vi "Create.vi"(7 "mode settings":variant, 8 "error in":errorcluster, 9 "number of channels":i32, 10 "channel settings":variant, 11 "digital output mode in":refnum<class "Digital Output Mode.lvclass">) -> (0 "error out":errorcluster, 1 "channels":refnum<class "Channel.lvclass">[](array[class]), 3 "digital output mode out":refnum<class "Digital Output Mode.lvclass">)   [LabVIEW 2017, in "Scan Engine Scripting.lvlib" / "Digital Output Mode.lvclass"]
uses:
  Digital Output Mode.lvclass
  Channel Classes/Channel/Channel.lvclass
  Controls/digital channel settings.ctl
  Channel Classes/DO Channel/DO Channel.lvclass
  C:/dev/github.com/debryant/niveristand-scan-engine-ethercat-custom-device/Custom Device Source/Scripting/Modules/Channel Classes/Channel/Channel.lvclass
  Scan Engine Scripting.lvlib
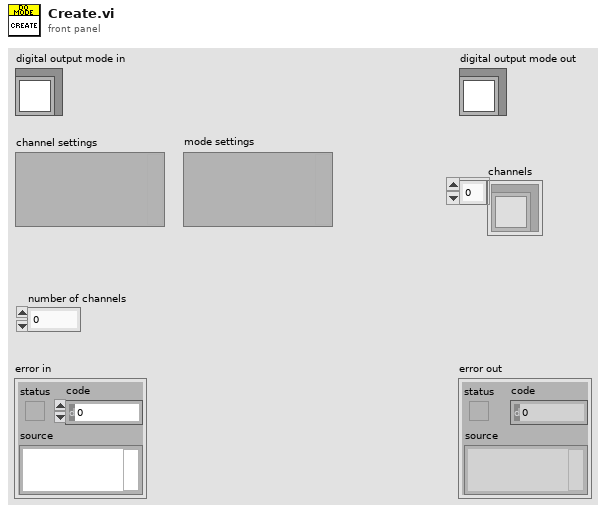
[diagram p1: front panel]
types:
  T1 = typedef "Scan Engine Scripting.lvlib/digital channel settings.ctl" = cluster{"name":string, "default value":bool}
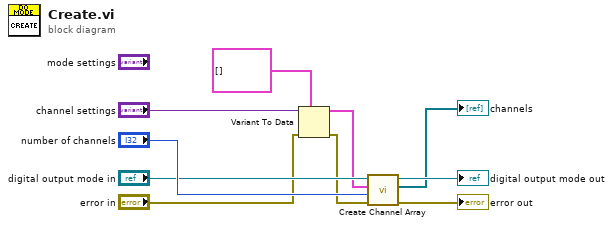
[diagram p0: block diagram]
diagram:
  n1 = Variant To Data(error in="error in", type=T1[] [] ("channel settings"), Variant="channel settings") -> (data=w3:T1[], error out=w2:errorcluster)
  n2 = call "Create Channel Array.vi"("error in"=w2, "expected channel count"="number of channels", "channel settings"=w3, "digital output mode in"="digital output mode in") -> ("error out"=→"error out":errorcluster, "channels"=→"channels":refnum<class "DO Channel.lvclass">[], "digital output mode out"=→"digital output mode out":refnum<class "Digital Output Mode.lvclass">)  [unwired: 5 in]
